vi "Converti AI.vi"(6 "Offset":dbl, 7 "Dato":dbl, 9 "Range":dbl, 10 "Ai_MAX":dbl, 11 "AI min":dbl) -> (3 "Dato convertito":dbl)   [LabVIEW 2019]
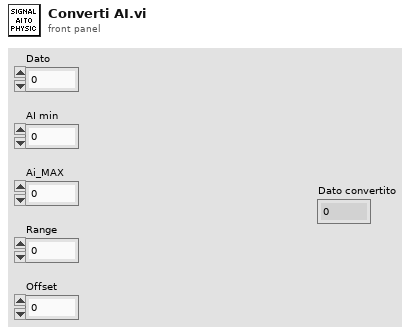
[diagram p1: front panel]
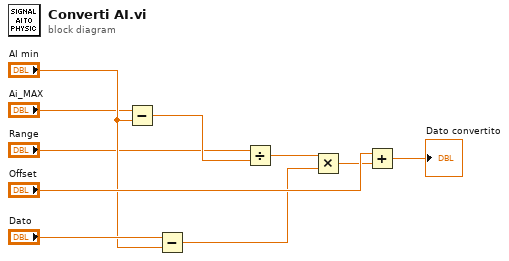
[diagram p0: block diagram]
diagram:
  n1 = Subtract(x="Ai_MAX", y="AI min") -> (x-y=w3:dbl)
  n2 = Subtract(x="Dato", y="AI min") -> (x-y=w6:dbl)
  n3 = Divide(x="Range", y=w3) -> (x/y=w5:dbl)
  n4 = Multiply(x=w5, y=w6) -> (x*y=w7:dbl)
  n5 = Add(x="Offset", y=w7) -> (x+y=→"Dato convertito":dbl)
